vi "uc480_SubVI_Example_GetPixelClock.vi"(0 ".NET (Reference)":refnum<k24>, 11 "Error In":errorcluster) -> (4 "Pixel Clock":i32, 6 "Inc":i32, 8 "Min":i32, 10 "Max":i32, 15 "error out":errorcluster caption="Error Out")   [LabVIEW 2021]
uses:
  C:/Program Files/Thorlabs/Scientific Imaging/ThorCam/uc480DotNet.dll
  Program Files/Thorlabs/Scientific Imaging/ThorCam/uc480DotNet.dll
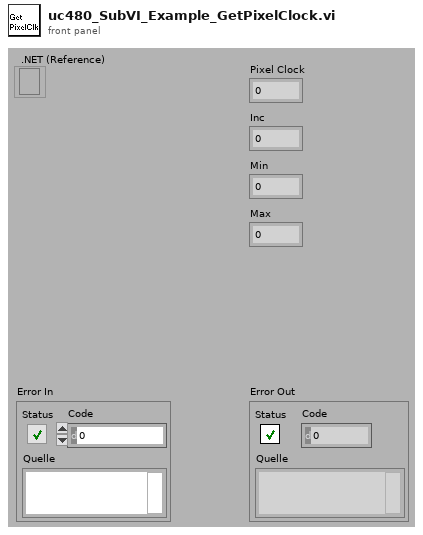
[diagram p1: front panel]
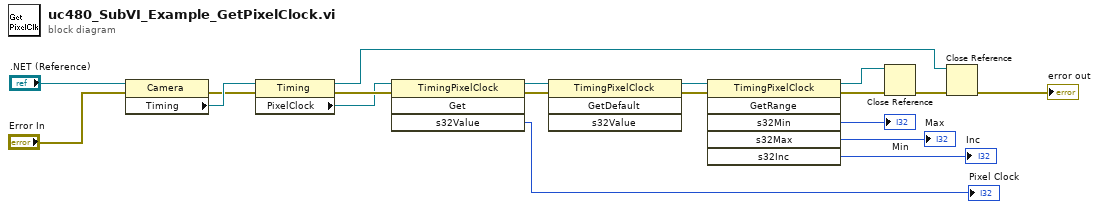
[diagram p0: block diagram]
diagram:
  n1 = property class="Camera"(reference=".NET (Reference)", error in="Error In") -> (error out=w18:errorcluster, "Timing"=w19:refnum<k24>)  [unwired: 1 out]
  n2 = property class="Timing"(reference=w19, error in=w18) -> (reference out=w5:refnum<k24>, error out=w17:errorcluster, "PixelClock"=w16:refnum<k24>)
  n3 = invoke class="TimingPixelClock" method="Get"(reference=w16, error in=w17) -> (reference out=w15:refnum<k24>, error out=w14:errorcluster, "s32Value"=→"Pixel Clock":i32)  [unwired: 2 in, 1 out]
  n4 = invoke class="TimingPixelClock" method="GetDefault"(reference=w15, error in=w14) -> (reference out=w12:refnum<k24>, error out=w13:errorcluster)  [unwired: 2 in, 2 out]
  n5 = invoke class="TimingPixelClock" method="GetRange"(reference=w12, error in=w13) -> (reference out=w4:refnum<k24>, error out=w3:errorcluster, "s32Min"=→"Min":i32, "s32Max"=→"Max":i32, "s32Inc"=→"Inc":i32)  [unwired: 4 in, 1 out]
  n6 = Close Reference(reference=w4, error in (no error)=w3) -> (error out=w1:errorcluster)
  n7 = Close Reference(reference=w5, error in (no error)=w1) -> (error out=→"error out":errorcluster)
